vi "LS218_01_alarm.vi"(3 "enabled":bool=TRUE, 5 "HIHI":dbl=1400.0 format="%.1f", 7 "HI":dbl=1300.0 format="%.1f", 8 "time_last_alarm_in":timestamp, 10 "readout_status":bool=TRUE, 11 "value_array":dbl[](array[numeric])) -> (0 "time_last_alarm_out":timestamp, 2 "alarm_status":u32(colorbox))   [LabVIEW 2019]
panel:
  out "message":string
  in  "interval":dbl=600.0
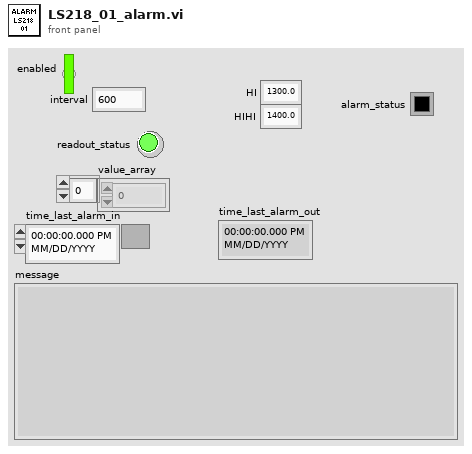
[diagram p1: front panel]
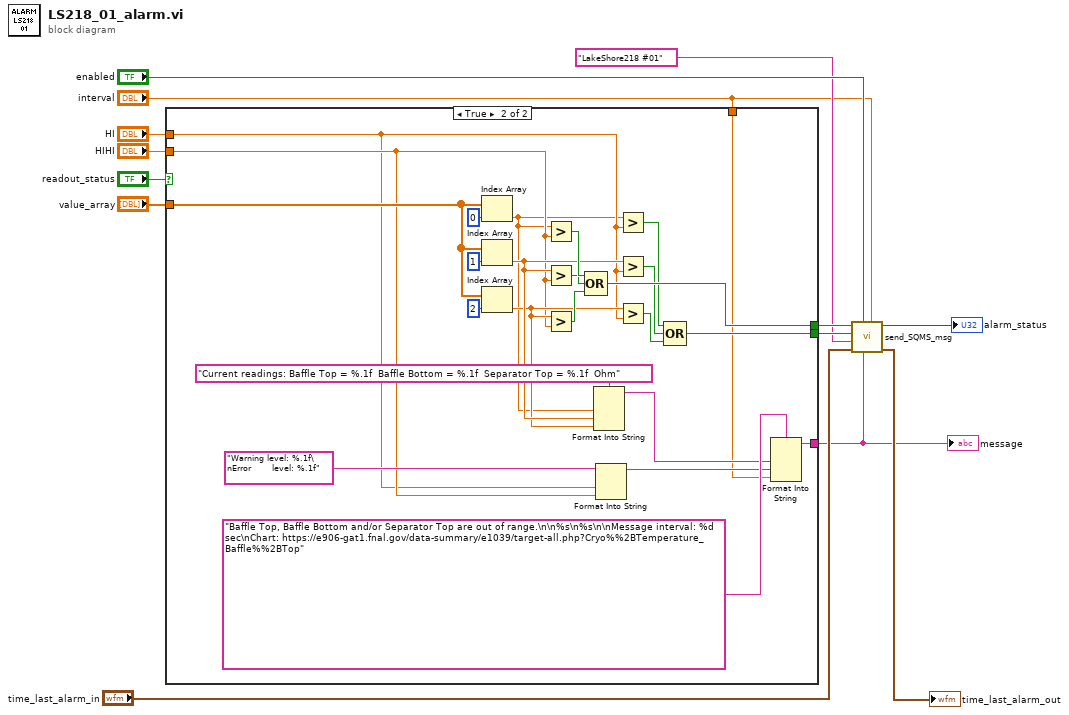
[diagram p0: block diagram]
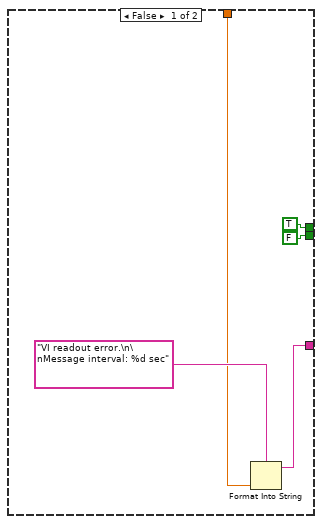
[diagram p2: hidden frame]
diagram:
  n1 = case shown="True" "readout_status" {
    tunnel: [TRUE w36] -> w12
    tunnel: [FALSE w32] -> w11
    tunnel: "value_array" -> [_ w30]
    tunnel: "HI" -> [_ w20]
    tunnel: "HIHI" -> [_ w21]
    tunnel: "interval" -> [w14 w23]
    tunnel: [w15 w22] -> w3
    frame False {
      n2 = Format Into String(format string="VI readout error.\n\nMessage interval: %d sec" ("msg"), w14) -> (resulting string=w15:string)  [unwired: 2 in, 1 out]
    }
    frame True {
      n3 = Index Array(array=w30, index=0) -> (element=w19:dbl)
      n4 = Index Array(array=w30, index=1) -> (element=w29:dbl)
      n5 = Index Array(array=w30, index=2) -> (element=w28:dbl)
      n6 = Greater?(x=w19, y=w21) -> (0:w39:bool)
      n7 = Greater?(x=w29, y=w21) -> (0:w38:bool)
      n8 = Greater?(x=w28, y=w21) -> (0:w37:bool)
      n9 = Compound Arithmetic op=OR(w39, w38, w37) -> (w36:bool)
      n10 = Format Into String(format string="Current readings: Baffle Top = %.1f  Baffle Bottom = %.1f  Separator Top = %.1f  Ohm" ("msg"), w19, w29, w28) -> (resulting string=w25:string)  [unwired: 2 in, 1 out]
      n11 = Format Into String(format string="Warning level: %.1f\nError       level: %.1f" ("msg"), w20, w21) -> (resulting string=w24:string)  [unwired: 2 in, 1 out]
      n12 = Greater?(x=w19, y=w20) -> (0:w35:bool)
      n13 = Greater?(x=w29, y=w20) -> (0:w34:bool)
      n14 = Greater?(x=w28, y=w20) -> (0:w33:bool)
      n15 = Compound Arithmetic op=OR(w35, w34, w33) -> (w32:bool)
      n16 = Format Into String(format string="Baffle Top, Baffle Bottom and/or Separator Top are out of range.\n\n%s\n%s\n\nMessage interval: %d sec\nChart: https://e906-gat1.fnal.gov/data-summary/e1039/target-all.php?Cryo%%2BTemperature_Baffle%%2BTop" ("msg"), w25, w24, w23) -> (resulting string=w22:string)  [unwired: 2 in, 1 out]
    }
  }
  "message" <- w3
  n17 = call "send_SQMS_msg.vi"("alarm_interval"="interval", "msg"=w3, "enabled"="enabled", "time_last_alarm_in"="time_last_alarm_in", "title"="LakeShore218 #01", "warning"=w11, "error"=w12) -> ("time_last_alarm_out"=→"time_last_alarm_out":timestamp, "alarm_status"=→"alarm_status":u32)  [unwired: 2 in, 1 out]
